vi "Read from File.vi"(8 "error in (no error)":errorcluster, 11 "Filename":string) -> (0 "error out":errorcluster, 1 "timed out?":bool, 2 "Message Data":variant, 3 "Message":string)   [LabVIEW 2015, in "Tool Interface.lvlib"]
uses:
  Tool Interface.lvlib
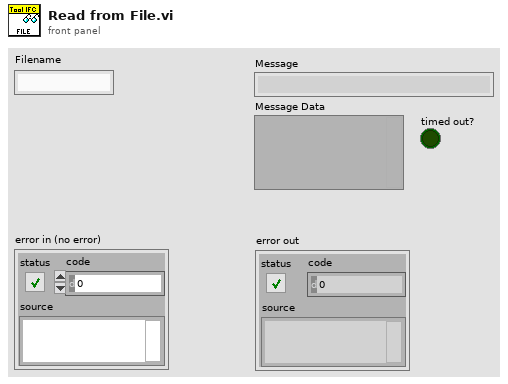
[diagram p1: front panel]
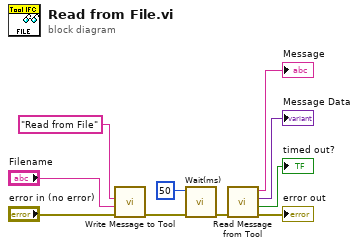
[diagram p0: block diagram]
diagram:
  n1 = call "Write Message to Tool.vi"("error in (no error)"="error in (no error)", "Message Data"="Filename", "Message"="Read from File") -> ("error out"=w10:errorcluster)  [unwired: 8 in]
  n2 = call "Wait(ms).vi"("error in (no error)"=w10, "milliseconds"=u32 50) -> ("error out"=w9:errorcluster)  [unwired: 9 in]
  n3 = call "Read Message from Tool.vi"("error in (no error)"=w9) -> ("error out"=→"error out":errorcluster, "timed out?"=→"timed out?":bool, "Message Data"=→"Message Data":variant, "Message"=→"Message":string)  [unwired: 7 in]
